vi "Vector2NumDen.vi"(11 "Filter Vector":dbl[](array[numeric])) -> (0 "Denominator":dbl[](array[numeric]), 1 "Numerator":dbl[](array[numeric]), 3 "FilterLength":i32)   [LabVIEW 2018, in "kevLib2010.lvlib"]
uses:
  kevLib2010.lvlib
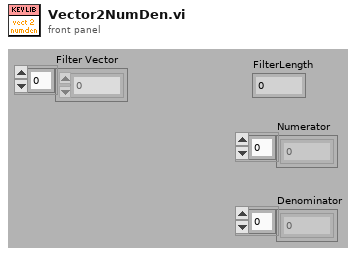
[diagram p1: front panel]
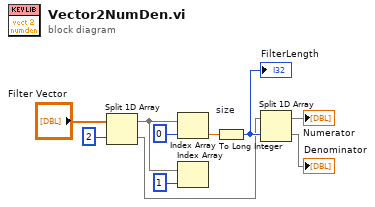
[diagram p0: block diagram]
diagram:
  n1 = Split 1D Array(array="Filter Vector", index=2) -> (first subarray=w5:dbl[], second subarray=w7:dbl[])
  n2 = Index Array(array=w5, index=0) -> (element=w6:dbl)
  n3 = Index Array(array=w5, index=1) -> ()  [unwired: 1 out]
  n4 = To Long Integer "size"(number=w6) -> (32bit integer=w8:i32)
  "FilterLength" <- w8
  n5 = Split 1D Array(array=w7, index=w8) -> (first subarray=→"Numerator":dbl[], second subarray=→"Denominator":dbl[])
